vi "Connect.vi"(8 "error in":errorcluster, 11 "2575 in":refnum<class "2575.lvclass">) -> (0 "error out":errorcluster, 3 "2575 out":refnum<class "2575.lvclass">)   [LabVIEW 2019, in "2575.lvlib" / "2575.lvclass"]
uses:
  Library/2575.lvclass
  C:/Users/Public/Documents/Development/builds/Instruments/Instruments.lvlibp/Library/Instruments.lvclass
  C:/Users/Public/Documents/Development/builds/Instruments/SwitchMatrix.lvlibp/Library/SwitchMatrix.lvclass
  Library/2575.lvclass/2575.ctl
  builds/Instruments/Instruments.lvlibp/Accessors/Read Simulated.vi
  builds/Instruments/Instruments.lvlibp/Accessors/Read Resource.vi
  builds/Instruments/SwitchMatrix.lvlibp/Accessors/Read Matrix Topology.vi
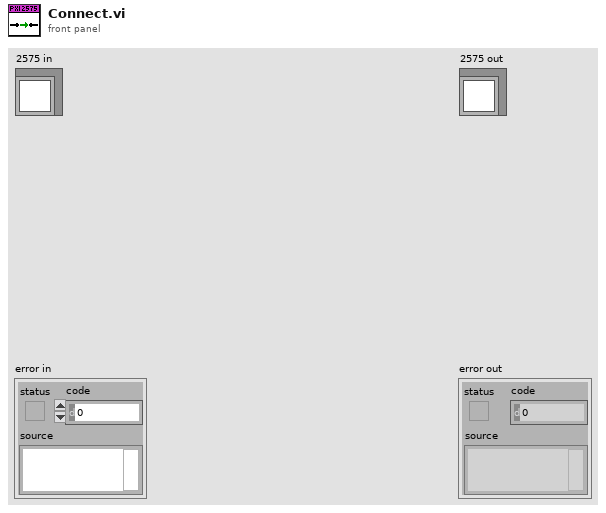
[diagram p1: front panel]
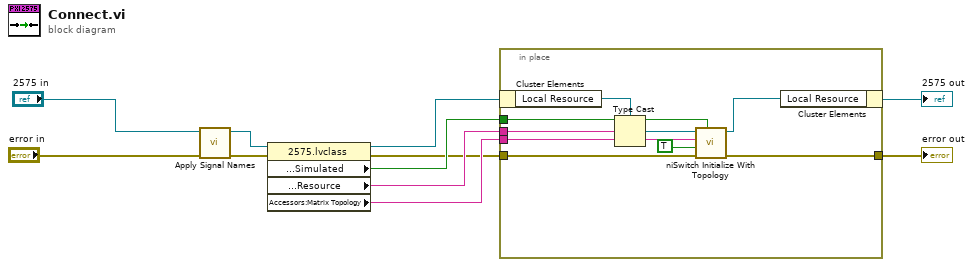
[diagram p0: block diagram]
diagram:
  n1 = call "Apply Signal Names.vi"("error in"="error in", "2575 in"="2575 in") -> ("error out"=w2:errorcluster, "2575 out"=w7:refnum<class "2575.lvclass">)  [unwired: 8 in]
  n2 = property class="2575.lvclass"(reference=w7, error in=w2) -> (reference out=w6:refnum<class "2575.lvclass">, error out=w1:errorcluster, "Accessors:Configuration:Simulated"=w5:bool, "Accessors:Configuration:Resource"=w4:string, "Accessors:Matrix Topology"=w3:string)
  n3 = in-place {
    in-place-border: w4 -> [w18]
    in-place-border: w3 -> [w16]
    in-place-border: w1 -> [w15]
    in-place-border: [w13] -> w10
    in-place-border: w5 -> [w12]
    n4 = in-place-cluster #1(w6) -> ("Local Resource"=w17:refnum<k15>)
    n5 = Type Cast(type=w17, x=w18) -> (*(type *) &x=w19:refnum<k15>)
    n6 = call <instrlib>:"niSwitch Initialize With Topology.vi"("simulate (boolean value)"=w12, "error in (no error)"=w15, "reset device (boolean value)"=TRUE ("simulate (boolean value)"), "topology name"=w16, "resource name"=w19) -> ("error out"=w13:errorcluster, "instrument handle out"=w14:refnum<k15>)  [unwired: 5 in]
    n7 = in-place-cluster #1("Local Resource"=w14) -> (→"2575 out":refnum<class "2575.lvclass">)
  }
  "error out" <- w10
